vi "Configure Load to Sequence-Ganging.vi"(8 "error in":errorcluster, 11 "Load to seq config - Ganging":T4={"Load Ganged Session Out"={"Ganged Config"=enum."Series", "Session List"=[], "Session Mode"=[], "Channel"=[]}, "Load sweep values"=[], "Source sweep points"=0, "Load output function"=1007, "Load transient response"=1038, "Load voltage/current gain bandwidth"=0.0, "Load voltage/current compensation frequency"=0.0, "Load voltage/current pole-zero ratio"=0.0, "Load aperture time"=0.0, "Load source delay"=0.0, "Load measure trigger"="", "Load source trigger"=""} {"Load transient response" items=["Slow"=1041, "Normal"=1038, "Fast"=1039, "Custom"=1042]; "Load output function" items=["DC Voltage"=1006, "DC Current"=1007, "Pulse Voltage"=1049, "Pulse Current"=1050]; "Load sweep values" format="%#_13g"}) -> (0 "error out":errorcluster, 3 "Ganged Session Out":T1)   [LabVIEW 2021]
doc: "This VI configures the ganged load to sequence mode."
uses:
  controls/Load to Sequence Config-Ganging.ctl
  channel ganging/shared subVIs/ctl/NIDCPower_channel_ganging - ctl - ganged config.ctl
  channel ganging/shared subVIs/ctl/NIDCPower_channel_ganging - ctl - channel mode.ctl
  channel ganging/shared subVIs/ctl/NIDCPower_channel_ganging - ctl - ganged session.ctl
  <instrlib>/niDCPower/nidcpower.llb/niDCPower Source Mode.ctl
  channel ganging/shared subVIs/Triggers and Events/NIDCPower_channel_ganging - Configure Digital Edge Source Trigger.vi
  channel ganging/shared subVIs/Triggers and Events/NIDCPower_channel_ganging - Disable Source Trigger.vi
  channel ganging/shared subVIs/Triggers and Events/NIDCPower_channel_ganging - Configure Digital Edge Measure Trigger.vi
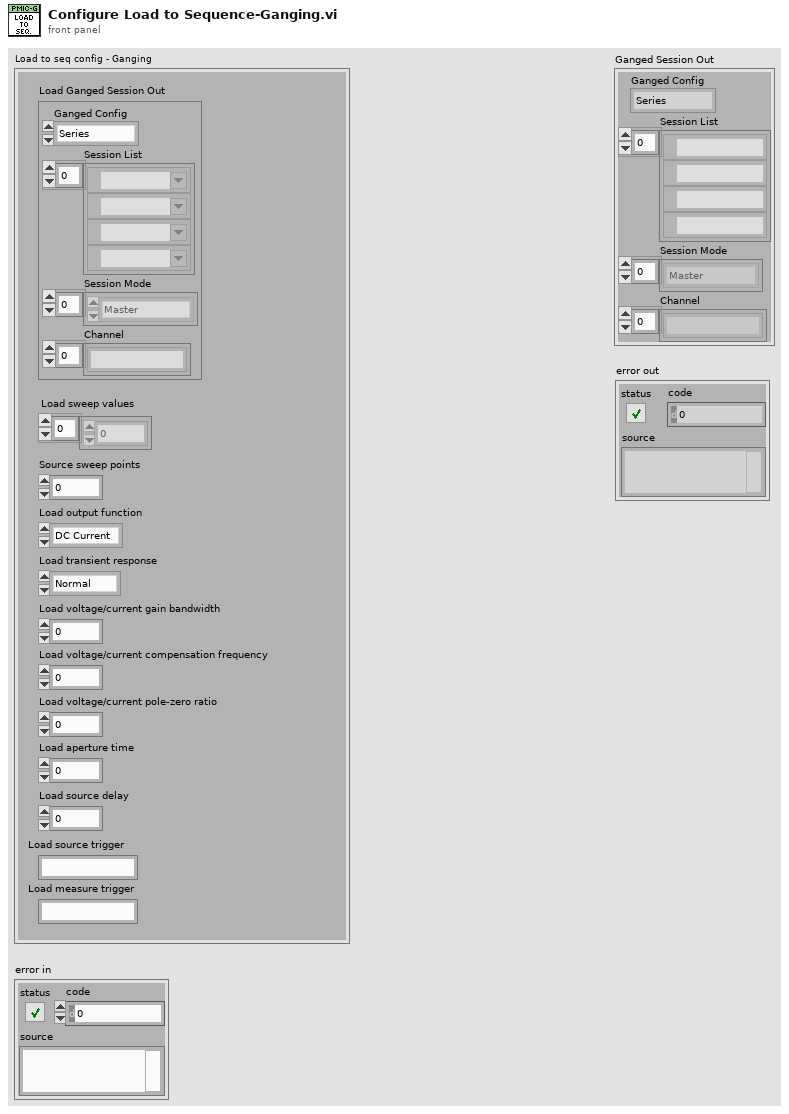
[diagram p1: front panel]
types:
  T1 = typedef "NIDCPower_channel_ganging - ctl - ganged session.ctl" = cluster{"Ganged Config":T2, "Session List":refnum<k15>[], "Session Mode":T3[], "Channel":string[]}
  T2 = typedef "NIDCPower_channel_ganging - ctl - ganged config.ctl" = enum32{"Series", "Parallel", "Manual"}
  T3 = typedef "NIDCPower_channel_ganging - ctl - channel mode.ctl" = enum32{"Master", "Slave", "Slave - Inverted"}
  T4 = typedef "Load to Sequence Config-Ganging.ctl" = cluster{"Load Ganged Session Out":cluster{"Ganged Config":T2, "Session List":refnum<k15>[], "Session Mode":T3[], "Channel":string[]}, "Load sweep values":dbl[], "Source sweep points":i32, "Load output function":i32, "Load transient response":i32, "Load voltage/current gain bandwidth":dbl, "Load voltage/current compensation frequency":dbl, "Load voltage/current pole-zero ratio":dbl, "Load aperture time":dbl, "Load source delay":dbl, "Load measure trigger":string, "Load source trigger":string}
  T5 = typedef "niDCPower Source Mode.ctl" = i32
  T6 = cluster{"Ganged Config":T2, "Session List":refnum<k15>[], "Session Mode":T3[], "Channel":string[]}
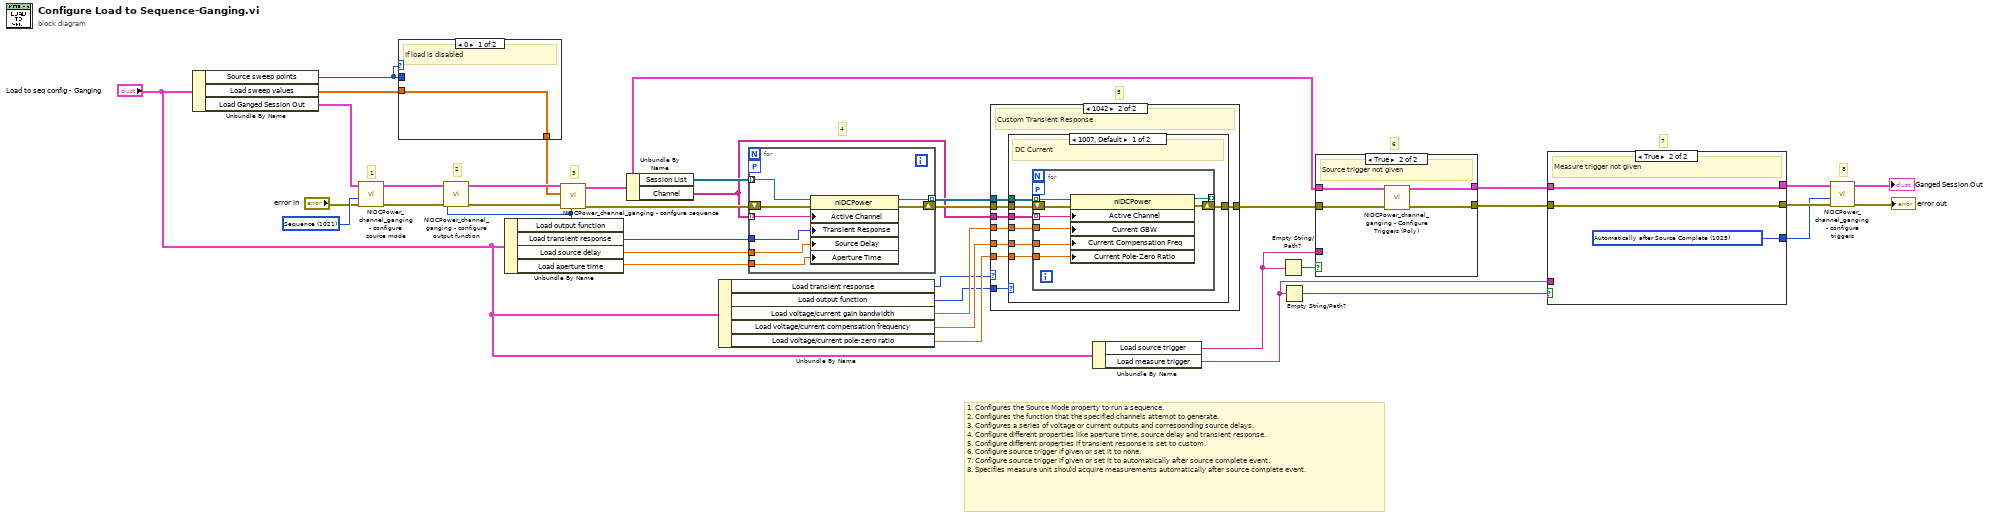
[diagram p0: block diagram]
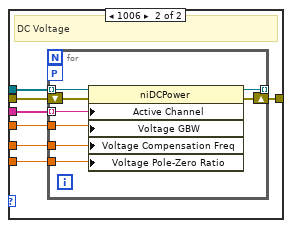
[diagram p3: hidden frame]
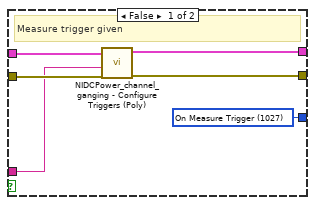
[diagram p5: hidden frame]
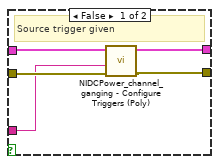
[diagram p6: hidden frame]
diagram:
  w36 = T5 1021 items=["Single Point"=1020, "Sequence"=1021] ("source mode")
  # "1. Configures the Source Mode property to run a sequence.\n2. Configures the function that the specified channels attempt to generate.\n3. Configures a series of voltage or current outputs and corresponding source delays. \n4. Configure different properties like aperture time, source delay and transient response.\n5. Configure different properties if transient response is set to custom.\n6. Configure source trigger if given or set it to none.\n7. Configure source trigger if given or set it to automatically after source complete event.\n8. Specifies measure unit should acquire measurements automatically after source complete event."
  # "8"
  # "7"
  # "6"
  # "5"
  # "4"
  # "3"
  # "2"
  # "1"
  n1 = Unbundle By Name("Load to seq config - Ganging") -> ("Source sweep points"=w19:i32, "Load sweep values"=w20:dbl[], "Load Ganged Session Out"=w21:T6)
  n2 = call "NIDCPower_channel_ganging - configure source mode.vi"("error in (no error)"="error in", "source mode"=w36, "Ganged Session In"=w21) -> ("error out"=w38:errorcluster, "Ganged Session Out"=w37:T1)  [unwired: 7 in]
  n3 = case shown="0" w19 {
    tunnel: [w39 w42] -> w22
    tunnel: w20 -> [w39 w41]
    tunnel: w19 -> [_ w40]
    frame 0 {
      # "If load is disabled"
    }
    frame 1, Default {
      # "If source is enabled"
      n4 = for {
        N: w40 -> [_]
        tunnel: w41 -> [w44]
        tunnel: [w43] -> w42 mode=concatenating
        n5 = for {
          tunnel: w44 -> [w45] mode=indexing
          tunnel: [w45] -> w43 mode=indexing
        }
      }
    }
  }
  n6 = Unbundle By Name("Load to seq config - Ganging") -> ("Load output function"=w11:i32, "Load transient response"=w7:i32, "Load source delay"=w26:dbl, "Load aperture time"=w25:dbl)
  n7 = call "NIDCPower_channel_ganging - configure output function.vi"("error in (no error)"=w38, "output function"=w11, "Ganged Session In"=w37) -> ("error out"=w34:errorcluster, "Ganged Session Out"=w35:T1)  [unwired: 7 in]
  n8 = call "NIDCPower_channel_ganging - confgure sequence.vi"("output function"=w11, "error in (no error)"=w34, "Values"=w22, "Ganged Session In"=w35) -> ("error out"=w33:errorcluster, "Ganged Session Out"=w8:T1)  [unwired: 6 in]
  n9 = Unbundle By Name(w8) -> ("Session List"=w32:refnum<k15>[], "Channel"=w15:string[])
  n10 = Unbundle By Name("Load to seq config - Ganging") -> ("Load transient response"=w2:i32, "Load output function"=w1:i32, "Load voltage/current gain bandwidth"=w14:dbl, "Load voltage/current compensation frequency"=w13:dbl, "Load voltage/current pole-zero ratio"=w12:dbl)
  n11 = for {
    tunnel: [w53] -> w17 mode=indexing
    shift-right: [w51] -> w18
    shift-left: w33 -> [w52]
    workers-P: _ -> [_]
    tunnel: w32 -> [w50] mode=indexing
    tunnel: w15 -> [w49] mode=indexing
    tunnel: w7 -> [w48]
    tunnel: w26 -> [w47]
    tunnel: w25 -> [w46]
    n12 = property class="niDCPower"(reference=w50, error in=w52, "Active Channel"=w49, "Transient Response"=w48, "Source Delay"=w47, "Aperture Time"=w46) -> (reference out=w53:refnum<k15>, error out=w51:errorcluster)
  }
  n13 = case shown="1042" w2 {
    tunnel: w18 -> [w54 w62]
    tunnel: w17 -> [_ w61]
    tunnel: [w54 w60] -> w16
    tunnel: w15 -> [_ w59]
    tunnel: w14 -> [_ w58]
    tunnel: w13 -> [_ w57]
    tunnel: w12 -> [_ w56]
    tunnel: w1 -> [_ w55]
    frame Default {
      # "Slow, Normal and Fast Transient Response"
    }
    frame 1042 {
      # "Custom Transient Response"
      n14 = case shown="1007, Default" w55 {
        tunnel: w62 -> [w69 w84]
        tunnel: [w68 w83] -> w60
        tunnel: w61 -> [w67 w82]
        tunnel: w59 -> [w65 w81]
        tunnel: w58 -> [w66 w80]
        tunnel: w56 -> [w63 w78]
        tunnel: w57 -> [w64 w79]
        frame 1007, Default {
          # "DC Current"
          n15 = for {
            workers-P: _ -> [_]
            shift-right: [w76] -> w68
            shift-left: w69 -> [w77]
            tunnel: w67 -> [w75] mode=indexing
            tunnel: [w74] -> _ mode=indexing
            tunnel: w66 -> [w73]
            tunnel: w65 -> [w72] mode=indexing
            tunnel: w64 -> [w71]
            tunnel: w63 -> [w70]
            n16 = property class="niDCPower"(reference=w75, error in=w77, "Active Channel"=w72, "Current GBW"=w73, "Current Compensation Freq"=w71, "Current Pole-Zero Ratio"=w70) -> (reference out=w74:refnum<k15>, error out=w76:errorcluster)
          }
        }
        frame 1006 {
          # "DC Voltage"
          n17 = for {
            workers-P: _ -> [_]
            shift-right: [w85] -> w83
            shift-left: w84 -> [w92]
            tunnel: w82 -> [w91] mode=indexing
            tunnel: [w90] -> _ mode=indexing
            tunnel: w81 -> [w89] mode=indexing
            tunnel: w80 -> [w88]
            tunnel: w79 -> [w87]
            tunnel: w78 -> [w86]
            n18 = property class="niDCPower"(reference=w91, error in=w92, "Active Channel"=w89, "Voltage GBW"=w88, "Voltage Compensation Freq"=w87, "Voltage Pole-Zero Ratio"=w86) -> (reference out=w90:refnum<k15>, error out=w85:errorcluster)
          }
        }
      }
    }
  }
  n19 = Unbundle By Name("Load to seq config - Ganging") -> ("Load source trigger"=w10:string, "Load measure trigger"=w9:string)
  n20 = Empty String/Path?(string/path=w10) -> (empty?=w24:bool)
  n21 = Empty String/Path?(string/path=w9) -> (empty?=w23:bool)
  n22 = case shown="True" w24 {
    tunnel: w16 -> [w97 w101]
    tunnel: [w96 w100] -> w29
    tunnel: [w95 w99] -> w28
    tunnel: w10 -> [w94 _]
    tunnel: w8 -> [w93 w98]
    frame False {
      # "Source trigger given"
      n23 = call-poly "NIDCPower_channel_ganging - Configure Triggers (Poly).vi"("error in (no error)"=w97, "output terminal"=w94, "Ganged Session in"=w93) -> ("error out"=w95:errorcluster, "Ganged Session out"=w96:T1)  [unwired: 7 in]
    }
    frame True {
      # "Source trigger not given"
      n24 = call-poly "NIDCPower_channel_ganging - Configure Triggers (Poly).vi"("error in (no error)"=w101, "Ganged Session in"=w98) -> ("error out"=w99:errorcluster, "Ganged Session out"=w100:T1)  [unwired: 8 in]
    }
  }
  n25 = case shown="True" w23 {
    tunnel: [w107 w109] -> w31
    tunnel: [w106 w108] -> w30
    tunnel: w29 -> [w105 w109]
    tunnel: w28 -> [w104 w108]
    tunnel: [w103 w110] -> w27
    tunnel: w9 -> [w102 _]
    frame False {
      w103 = 1027 items=["Automatically after Source Complete"=1025, "On Demand"=1026, "On Measure Trigger"=1027] ("Measure When")
      # "Measure trigger given"
      n26 = call-poly "NIDCPower_channel_ganging - Configure Triggers (Poly).vi"("error in (no error)"=w104, "output terminal"=w102, "Ganged Session in"=w105) -> ("error out"=w106:errorcluster, "Ganged Session out"=w107:T1)  [unwired: 7 in]
    }
    frame True {
      w110 = 1025 items=["Automatically after Source Complete"=1025, "On Demand"=1026, "On Measure Trigger"=1027] ("Measure When")
      # "Measure trigger not given"
    }
  }
  n27 = call "NIDCPower_channel_ganging - configure triggers.vi"("error in (no error)"=w30, "Measure When"=w27, "Ganged Session In"=w31) -> ("error out"=→"error out":errorcluster, "Ganged Session Out"=→"Ganged Session Out":T1)  [unwired: 7 in]
